vi "HexToFloat.vi"(11 "数组":u16[](array[numeric]) format="%04xH") -> (3 "FLOAT":sgl[](array[numeric]))   [LabVIEW 2016, in "斯坦道总磷总氮.lvlib"]
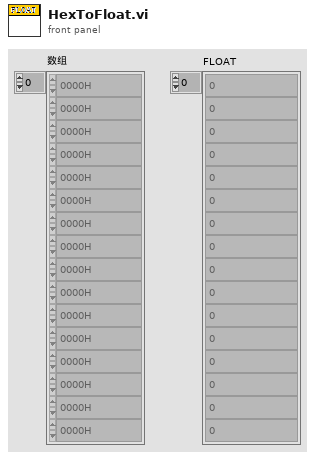
[diagram p1: front panel]
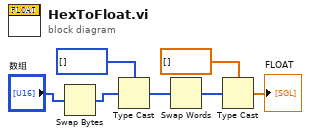
[diagram p0: block diagram]
diagram:
  n1 = Swap Bytes(anything="数组") -> (byte swapped=w1:u16[])
  n2 = Type Cast(type=u32[] [], x=w1) -> (*(type *) &x=w4:u32[])
  n3 = Swap Words(1:w4) -> (0:w3:u32[])
  n4 = Type Cast(type=sgl[] [], x=w3) -> (*(type *) &x=→"FLOAT":sgl[])
